vi "Periodic Tasks.vi"() -> ()   [LabVIEW 2018]
doc: "This VI runs in parallel to other tasks. It can contain as many user-defined periodic loops as you need. These can carry out PID or other sorts of timed response."
uses:
  Robot Global Data.vi
panel:
  out "new value":bool
  out "STEAK":dbl
  out "SCORE":dbl
  out "Collector Angle:\nWHOP on FLOOR":bool
  out "Collector Angle Down/Out":bool
  out "Kick Hatch":bool
  out "Hatch Retainer\nOpen/Close":bool
  out "HAB 3:\nFront Cylinders Only":bool
  out "HAB 3:\nDrive Module Forward":bool
  out "HAB 3:\nBack Cylinders Only":bool
  out "HAB 3:\nAll Cylinders":bool
  out "HAB 3:\nOverride Switches":bool
  out "Collector Angle:\nVertical":bool
  out "Collector Angle In":bool
  out "wrong answer":bool
  in  "error in":errorcluster
  # "do not touch dis"
  # "HERE IT IS AGAIN IN CASE U NEED IT!!!"
  # "HOW TO RUN GAME:"
  # "1.) In the bottom left corner, there is a white box \n     that says \"2019 Aux Game V.3.0.lvproj/Target\"\n     Right-click this and click\n     \"2019 Aux Game V.3.0.lvproj/My Computer\"\n2.) Run the code by pressing CTRL+R\n      Wait for everything to load and ignore the FRC Simulation\n4.) In Robot Main, press CTRL+E to open the block diagram\n5.) Press the VI that had Timed Tasked in the icon (it is labeled)\n======THIS IS THE GAME SCREEN!!========\n6.) Open the drivers station, plug in the aux controller\n7.) Click enable and go back to the Periodic Tasks \n      Front Panel to play!!"
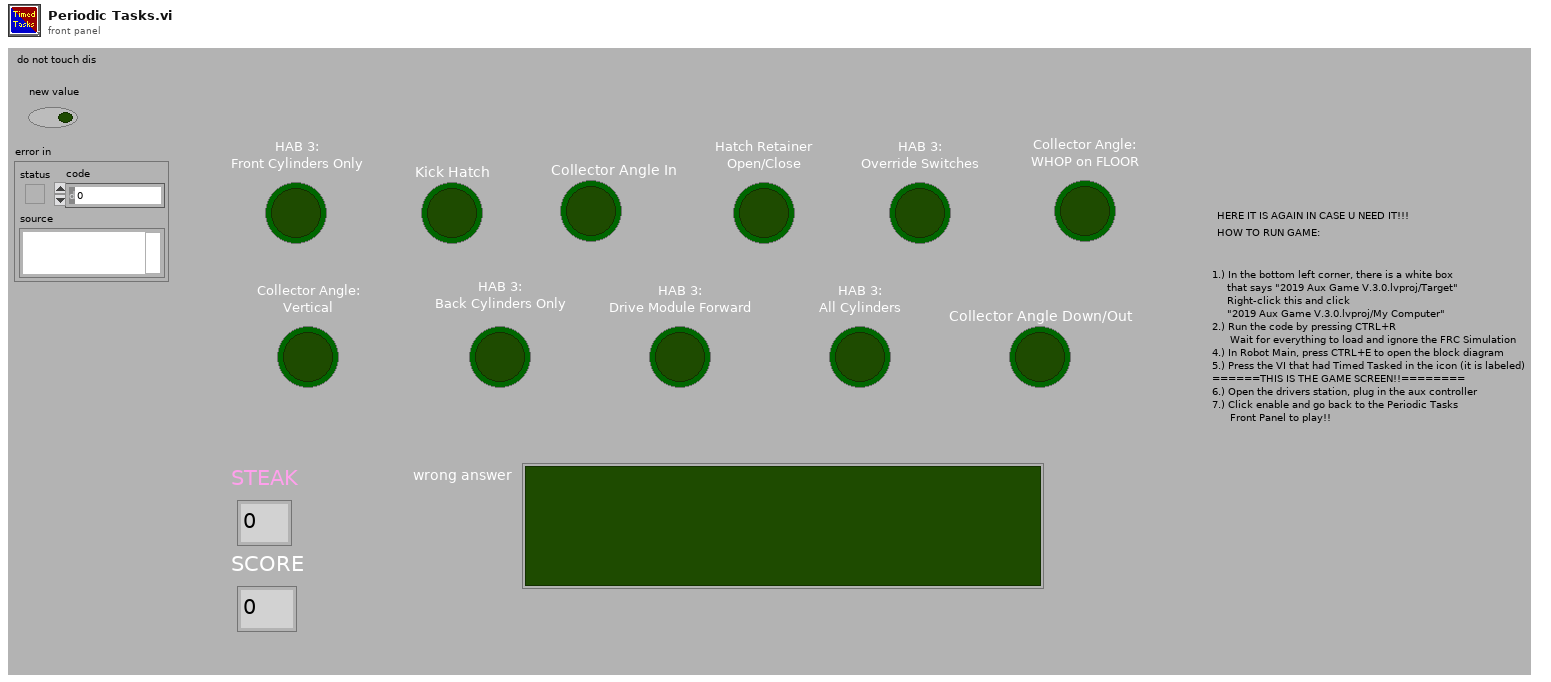
[diagram p1: front panel]
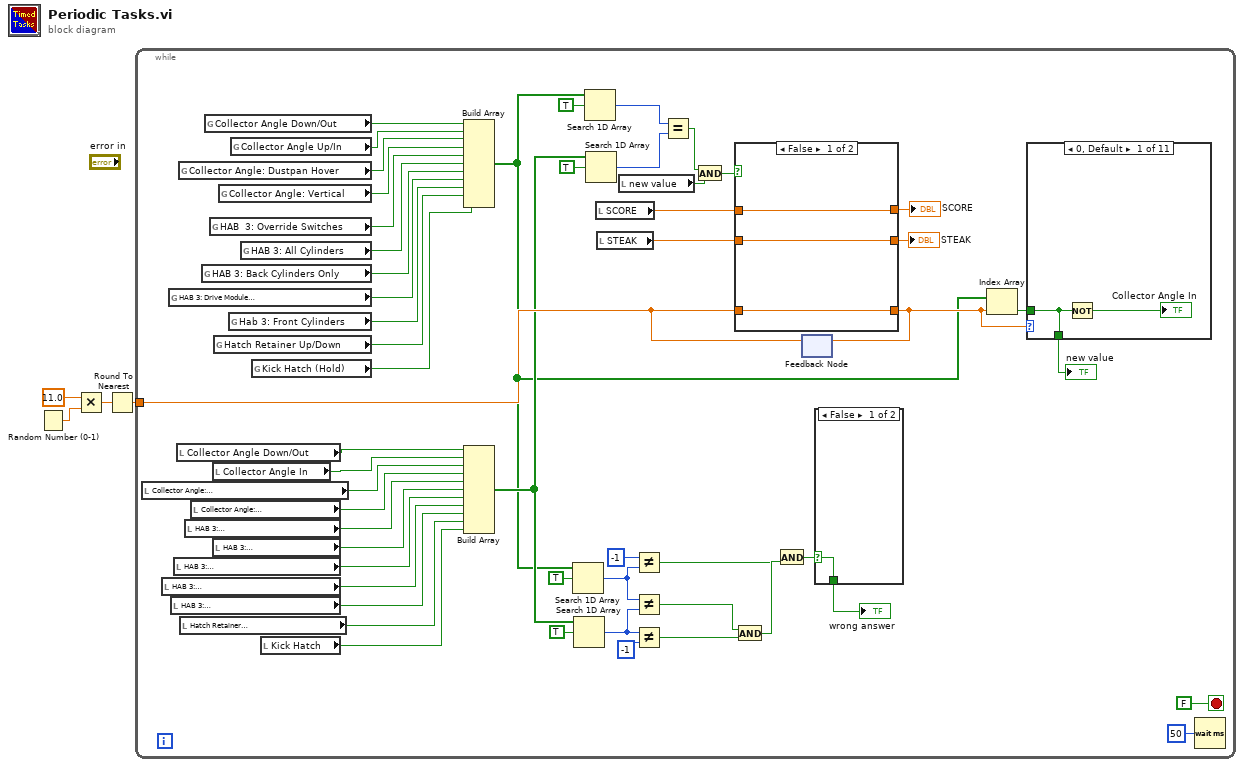
[diagram p0: block diagram]
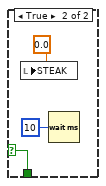
[diagram p2: hidden frame]
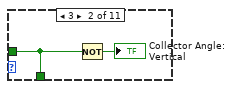
[diagram p3: hidden frame]
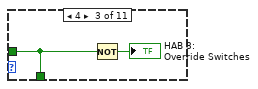
[diagram p4: hidden frame]
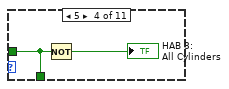
[diagram p5: hidden frame]
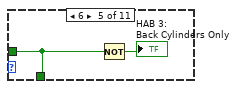
[diagram p6: hidden frame]
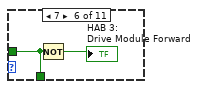
[diagram p7: hidden frame]
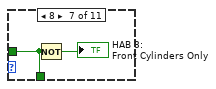
[diagram p8: hidden frame]
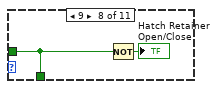
[diagram p9: hidden frame]
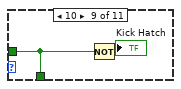
[diagram p10: hidden frame]
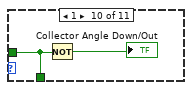
[diagram p11: hidden frame]
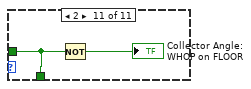
[diagram p12: hidden frame]
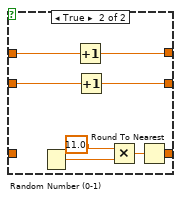
[diagram p13: hidden frame]
diagram:
  n1 = Random Number (0-1)() -> (number: 0 to 1=w4:dbl)
  n2 = Multiply(x=11.0, y=w4) -> (x*y=w2:dbl)
  n3 = Round To Nearest(number=w2) -> (nearest integer value=w1:dbl)
  n4 = while {
    tunnel: [w16] -> _
    tunnel: w1 -> [_]
    stop <- FALSE stop-if-true
    n5 = local read "Collector Angle:\nWHOP on FLOOR"() -> (w25:bool)
    n6 = local read "HAB 3:\nDrive Module Forward"() -> (w20:bool)
    n7 = global read "Robot Global Data.vi" "HAB 3: Drive Module\n(FORWARD)"() -> (w50:bool)
    n8 = local read "HAB 3:\nFront Cylinders Only"() -> (w19:bool)
    n9 = local read "HAB 3:\nBack Cylinders Only"() -> (w21:bool)
    n10 = local read "Collector Angle Down/Out"() -> (w27:bool)
    n11 = global read "Robot Global Data.vi" "Collector Angle: Dustpan Hover"() -> (w55:bool)
    n12 = local read "Hatch Retainer\nOpen/Close"() -> (w18:bool)
    n13 = local read "HAB 3:\nOverride Switches"() -> (w23:bool)
    n14 = local read "Collector Angle:\nVertical"() -> (w24:bool)
    n15 = global read "Robot Global Data.vi" "HAB 3: Back Cylinders Only"() -> (w51:bool)
    n16 = global read "Robot Global Data.vi" "Collector Angle Down/Out"() -> (w57:bool)
    n17 = global read "Robot Global Data.vi" "HAB  3: Override Switches"() -> (w53:bool)
    n18 = local read "Collector Angle In"() -> (w26:bool)
    n19 = local read "HAB 3:\nAll Cylinders"() -> (w22:bool)
    n20 = global read "Robot Global Data.vi" "Hatch Retainer Up/Down"() -> (w48:bool)
    n21 = global read "Robot Global Data.vi" "Collector Angle: Vertical"() -> (w54:bool)
    n22 = global read "Robot Global Data.vi" "Hab 3: Front Cylinders"() -> (w49:bool)
    n23 = global read "Robot Global Data.vi" "Collector Angle Up/In"() -> (w56:bool)
    n24 = global read "Robot Global Data.vi" "HAB 3: All Cylinders"() -> (w52:bool)
    n25 = global read "Robot Global Data.vi" "Kick Hatch (Hold)"() -> (w47:bool)
    n26 = local read "Kick Hatch"() -> (w17:bool)
    n27 = Build Array(w57, w56, w55, w54, w53, w52, w51, w50, w49, w48, w47) -> (w11:bool[])
    n28 = Build Array(w27, w26, w25, w24, w23, w22, w21, w20, w19, w18, w17) -> (w13:bool[])
    n29 = Search 1D Array(1D array=w11, element=TRUE) -> (index of element=w32:i32)  [unwired: 1 in]
    n30 = Search 1D Array(1D array=w13, element=TRUE) -> (index of element=w35:i32)  [unwired: 1 in]
    n31 = Search 1D Array(1D array=w11, element=TRUE) -> (index of element=w10:i32)  [unwired: 1 in]
    n32 = Search 1D Array(1D array=w13, element=TRUE) -> (index of element=w9:i32)  [unwired: 1 in]
    n33 = local read "SCORE"() -> (w45:dbl)
    n34 = local read "STEAK"() -> (w42:dbl)
    n35 = local read "new value"() -> (w7:bool)
    n36 = Not Equal?(x=-1, y=w32) -> (x != y?=w30:bool)
    n37 = Not Equal?(x=w32, y=w35) -> (x != y?=w37:bool)
    n38 = Not Equal?(x=w35, y=-1 ("x")) -> (x != y?=w38:bool)
    n39 = Equal?(x=w10, y=w9) -> (x = y?=w6:bool)
    n40 = And(x=w6, y=w7) -> (x .and. y?=w5:bool)
    n41 = And(x=w37, y=w38) -> (x .and. y?=w33:bool)
    n42 = And(x=w30, y=w33) -> (x .and. y?=w39:bool)
    n43 = feedback #1() -> (w16:dbl)  [unwired: 1 in]
    n44 = case shown="False" w5 {
      tunnel: w45 -> [w86 w94]
      tunnel: [w86 w93] -> w44
      tunnel: [w85 w91] -> w43
      tunnel: w42 -> [w85 w92]
      tunnel: w16 -> [w84 _]
      tunnel: [w84 w87] -> w28
      frame False {
      }
      frame True {
        n45 = Random Number (0-1)() -> (number: 0 to 1=w90:dbl)
        n46 = Increment(x=w94) -> (x+1=w93:dbl)
        n47 = Increment(x=w92) -> (x+1=w91:dbl)
        n48 = Multiply(x=11.0, y=w90) -> (x*y=w88:dbl)
        n49 = Round To Nearest(number=w88) -> (nearest integer value=w87:dbl)
      }
    }
    "STEAK" <- w43
    "SCORE" <- w44
    n50 = feedback-in #1(w28) -> ()
    n51 = case shown="False" w39 {
      selector: w39 -> [w58 w59]
      tunnel: [w58 w59] -> w29
      frame False {
      }
      frame True {
        n52 = local write "STEAK"(0.0) -> ()
        n53 = Wait (ms)(milliseconds to wait=u32 10) -> ()  [unwired: 1 out]
      }
    }
    "wrong answer" <- w29
    n54 = Index Array(array=w11, index=w28) -> (element=w15:bool)
    n55 = case shown="0, Default" w28 {
      tunnel: w15 -> [w62 w64 w66 w68 w70 w72 w74 w76 w78 w80 w82]
      tunnel: [w62 w64 w66 w68 w70 w72 w74 w76 w78 w80 w82] -> w8
      frame 0, Default {
        n56 = Not(x=w62) -> (.not. x?=→"Collector Angle In":bool)
      }
      frame 3 {
        n57 = Not(x=w64) -> (.not. x?=→"Collector Angle:\nVertical":bool)
      }
      frame 4 {
        n58 = Not(x=w66) -> (.not. x?=→"HAB 3:\nOverride Switches":bool)
      }
      frame 5 {
        n59 = Not(x=w68) -> (.not. x?=→"HAB 3:\nAll Cylinders":bool)
      }
      frame 6 {
        n60 = Not(x=w70) -> (.not. x?=→"HAB 3:\nBack Cylinders Only":bool)
      }
      frame 7 {
        n61 = Not(x=w72) -> (.not. x?=→"HAB 3:\nDrive Module Forward":bool)
      }
      frame 8 {
        n62 = Not(x=w74) -> (.not. x?=→"HAB 3:\nFront Cylinders Only":bool)
      }
      frame 9 {
        n63 = Not(x=w76) -> (.not. x?=→"Hatch Retainer\nOpen/Close":bool)
      }
      frame 10 {
        n64 = Not(x=w78) -> (.not. x?=→"Kick Hatch":bool)
      }
      frame 1 {
        n65 = Not(x=w80) -> (.not. x?=→"Collector Angle Down/Out":bool)
      }
      frame 2 {
        n66 = Not(x=w82) -> (.not. x?=→"Collector Angle:\nWHOP on FLOOR":bool)
      }
    }
    "new value" <- w8
    n67 = Wait (ms)(milliseconds to wait=u32 50) -> ()  [unwired: 1 out]
  }
